vi "Set Test Node Type.vi"(8 "error in (no error)":errorcluster, 10 "Test Node Type":string, 11 "Create Test Channel Model in":refnum<class "Create Test Channel Model.lvclass">) -> (0 "error out":errorcluster, 3 "Create Test Channel Model out":refnum<class "Create Test Channel Model.lvclass">)   [LabVIEW 2013, in "Create Test Channel Model.lvlib" / "Create Test Channel Model.lvclass"]
uses:
  Create Test Channel Model.lvclass
  Create Test Channel Model.lvclass/Create Test Channel Model.ctl
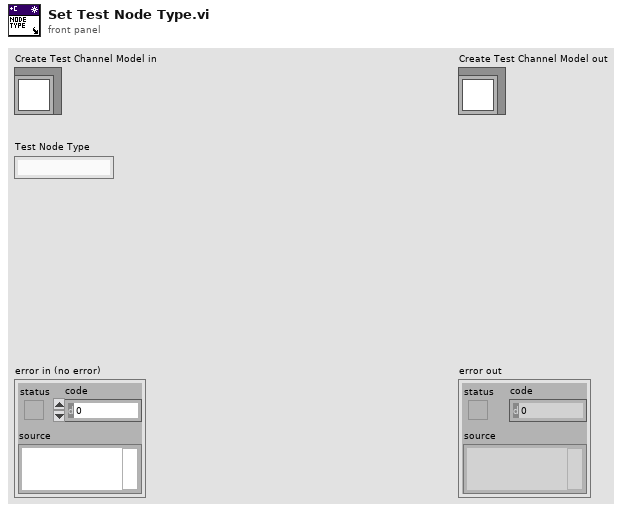
[diagram p1: front panel]
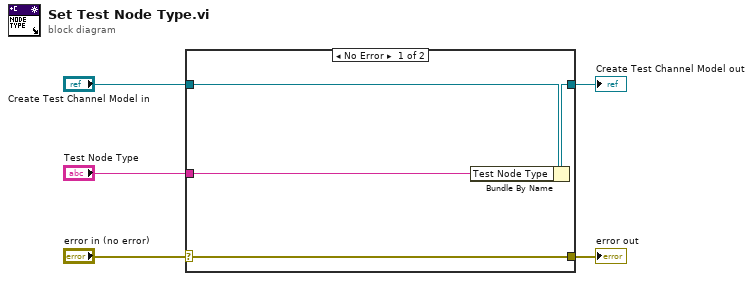
[diagram p0: block diagram]
diagram:
  n1 = case shown="No Error" "error in (no error)" {
    selector: "error in (no error)" -> [w9 w10]
    tunnel: [w9 w10] -> w4
    tunnel: [w7 w11] -> w2
    tunnel: "Create Test Channel Model in" -> [w8 w11]
    tunnel: "Test Node Type" -> [w6 _]
    frame No Error {
      n2 = Bundle By Name(cluster=w8, "Test Node Type"=w6) -> (w7:refnum<class "Create Test Channel Model.lvclass">)
    }
    frame Error {
    }
  }
  "error out" <- w4
  "Create Test Channel Model out" <- w2
